vi "Write Bacta [l].vi"(8 "error in (no error)":errorcluster, 10 "Bacta [l]":u8 max=100, 11 "BactaTank in":refnum<class "BactaTank.lvclass">) -> (0 "error out":errorcluster, 3 "BactaTank out":refnum<class "BactaTank.lvclass">)   [LabVIEW 2021, in "BactaTank.lvclass"]
uses:
  BactaTank.lvclass
  BactaTank.lvclass/BactaTank.ctl
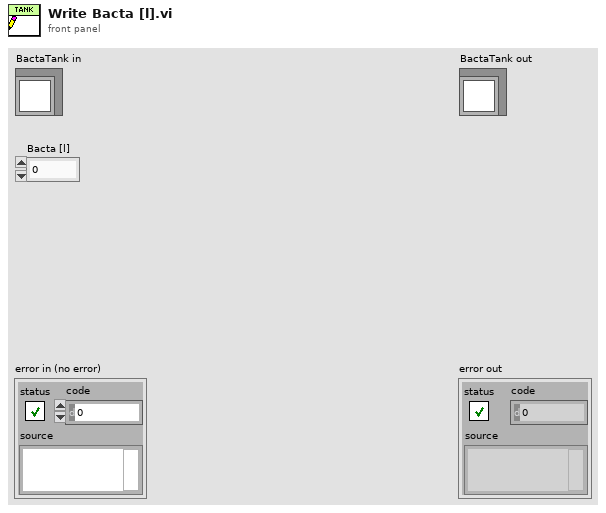
[diagram p1: front panel]
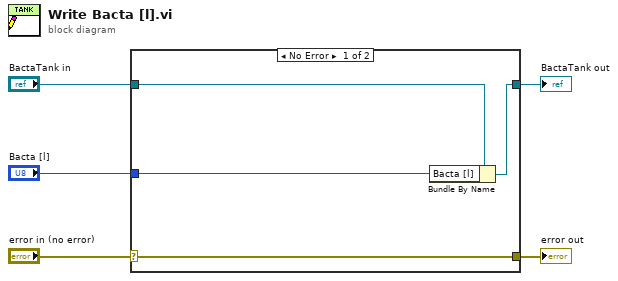
[diagram p0: block diagram]
diagram:
  n1 = case shown="No Error" "error in (no error)" {
    selector: "error in (no error)" -> [w9 w10]
    tunnel: [w9 w10] -> w4
    tunnel: [w7 w11] -> w2
    tunnel: "BactaTank in" -> [w8 w11]
    tunnel: "Bacta [l]" -> [w6 _]
    frame No Error {
      n2 = Bundle By Name(cluster=w8, "Bacta [l]"=w6) -> (w7:refnum<class "BactaTank.lvclass">)
    }
    frame Error {
    }
  }
  "error out" <- w4
  "BactaTank out" <- w2
